vi "Write Delimited Spreadsheet (string).vi"(0 "file path (dialog if empty)":path, 1 "format (%s)":string="%s", 5 "2D data":string[][](array[string]), 7 "1D data":string[](array[string]), 9 "append to file? (new file:F)":bool, 11 "error in (no error)":errorcluster, 12 "transpose? (no:F)":bool, 13 "delimiter (\\t)":string="\t") -> (4 "new file path (Not A Path if cancelled)":path, 15 "error out":errorcluster)   [LabVIEW 2018]
doc: "Converts a 2D or 1D array of strings, signed integers, or double-precision numbers to a text string and writes the string to a new byte stream file or appends the string to an existing file. Wire data to the <B>2D data</B> input or <B>1D data</B> input to determine the polymorphic instance to use or manually select the instance.\n\nUse this VI to transpose or separate data.\n\n<B>Note</B> To format with Microsoft Excel, use ActiveX with LabVIEW or the Report Generation Toolkit for Microsoft Office."
panel:
  in  "prompt":string="Choose file to write."
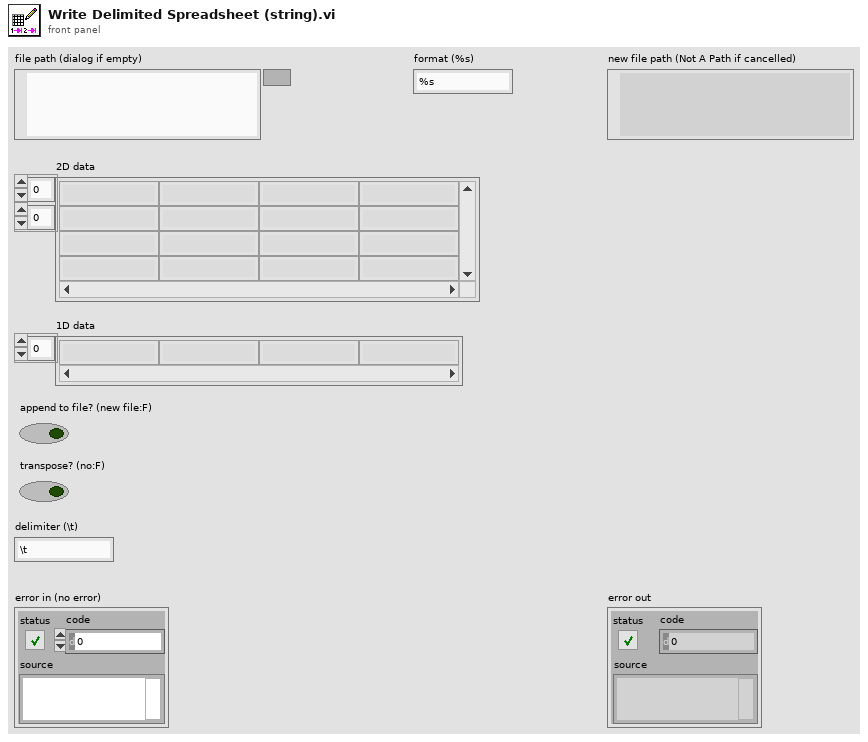
[diagram p1: front panel]
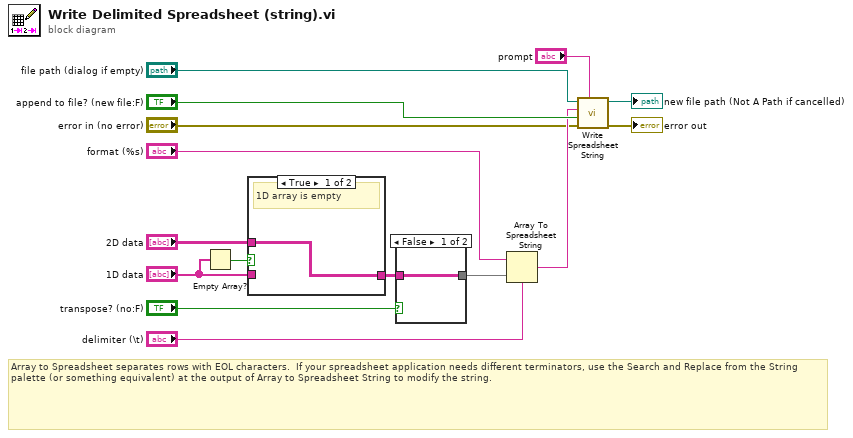
[diagram p0: block diagram]
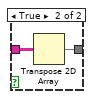
[diagram p2: hidden frame]
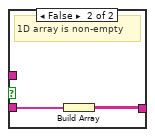
[diagram p3: hidden frame]
diagram:
  # "Array to Spreadsheet separates rows with EOL characters.  If your spreadsheet application needs different terminators, use the Search and Replace from the String palette (or something equivalent) at the output of Array to Spreadsheet String to modify the string."
  n1 = Empty Array?(array="1D data") -> (empty?=w15:bool)
  n2 = case shown="True" w15 {
    tunnel: "1D data" -> [_ w18]
    tunnel: [w16 w17] -> w11
    tunnel: "2D data" -> [w16 _]
    frame True {
      # "1D array is empty"
    }
    frame False {
      # "1D array is non-empty"
      n3 = Build Array(w18) -> (w17:string[][])
    }
  }
  n4 = case shown="False" "transpose? (no:F)" {
    tunnel: [w19 w21] -> w9
    tunnel: w11 -> [w19 w20]
    frame False {
    }
    frame True {
      n5 = Transpose 2D Array(2D array=w20) -> (transposed array=w21:string[][])
    }
  }
  n6 = Array To Spreadsheet String(delimiter (Tab)="delimiter (\\t)", array=w9, 3:"format (%s)") -> (spreadsheet string=w3:string)
  n7 = call "Write Spreadsheet String.vi"("prompt"="prompt", "error in"="error in (no error)", "append to file? (new file:F)"="append to file? (new file:F)", "spreadsheet string"=w3, "file path (dialog if empty)"="file path (dialog if empty)") -> ("error out"=→"error out":errorcluster, "path"=→"new file path (Not A Path if cancelled)":path)  [unwired: 5 in]
